vi "N5700 Config Current Limit.vi"(5 "error":errorcluster, 6 "Settle (0 mS)":u32, 7 "Current Limit":dbl format="%.4f", 8 "VISA":refnum<visa-resource-name>) -> (0 "error out":errorcluster, 3 "VISA out":refnum<visa-resource-name>)   [LabVIEW 2020]
doc: "This VI sets the current limit (command \"CURR nn\"). The power supply output will go to this limit if the load causes Constant-Current operation.\n\nThis VI will wait for \"Settle\" milliseconds after setting the limit to allow the output to reach the new setting. If unwired, there will be no delay"
panel:
  # "Agilent Technologies  \nSeries N5700A\n  DC Power Supplies"
  # "Set the Current Limit"
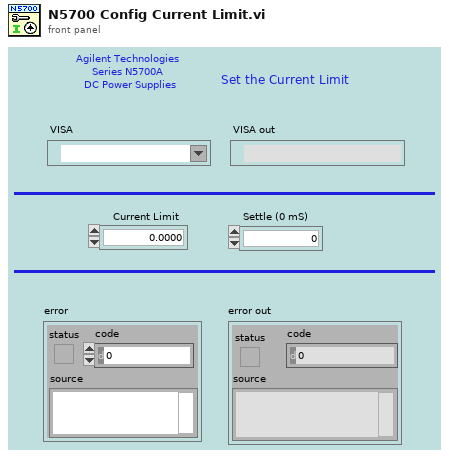
[diagram p1: front panel]
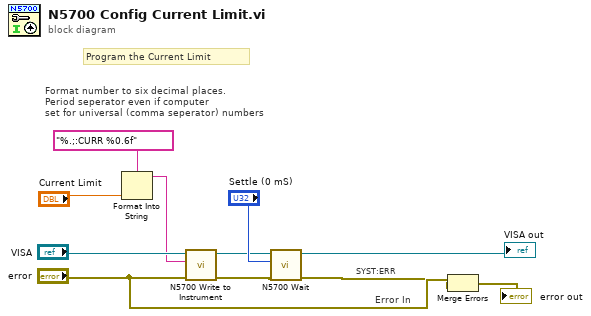
[diagram p0: block diagram]
diagram:
  # "SYST:ERR"
  # "Error In"
  # "Format number to six decimal places.\nPeriod seperator even if computer \nset for universal (comma seperator) numbers"
  # "Program the Current Limit"
  n1 = Format Into String(format string="%.;:CURR %0.6f", "Current Limit") -> (resulting string=w8:string)  [unwired: 2 in, 1 out]
  n2 = call "N5700 Write to Instrument.vi"("error"="error", "Command"=w8, "VISA"="VISA") -> ("error out"=w3:errorcluster, "VISA out"=w4:refnum<visa-resource-name>)  [unwired: 4 in]
  n3 = call "N5700 Wait.vi"("error"=w3, "Delay (5 mS)"="Settle (0 mS)", "VISA"=w4) -> ("error out"=w1:errorcluster, "VISA out"=→"VISA out":refnum<visa-resource-name>)  [unwired: 4 in]
  n4 = Merge Errors("error", w1) -> (→"error out":errorcluster)
